vi "Flatten.vi"(6 "Persistence in":refnum<class "IPersist.lvclass">, 7 "Linked List Ref":refnum<data-value>, 8 "error in (no error)":errorcluster, 9 "Indent":i32, 10 "Active Unique ID":string, 11 "Executioner in":refnum<class "Executioner.lvclass">) -> (0 "error out":errorcluster, 2 "Active Unique ID out":string, 3 "Flattened Test Executive":string[](array[string]), 4 "Persistence out":refnum<class "IPersist.lvclass">, 5 "Linked List Ref out":refnum<data-value>)   [LabVIEW 2017, in "Test Executive.lvlib" / "Executioner.lvclass"]
uses:
  <vilib>/gpm_packages/@cs/test-executive/Source/Test Executive/Executioner/Executioner.lvclass
  <vilib>/gpm_packages/@cs/linked-list/Source/Linked List/ILinkedList/ILinked List.lvclass
  <vilib>/gpm_packages/@cs/persistence/source/IPersist/IPersist.lvclass
  <vilib>/gpm_packages/@cs/linked-list/Source/Linked List/Linked List Ref/Linked List Ref.lvclass
  <vilib>/gpm_packages/@cs/linked-list/Source/String Manipulation/String Manipulation.lvlib
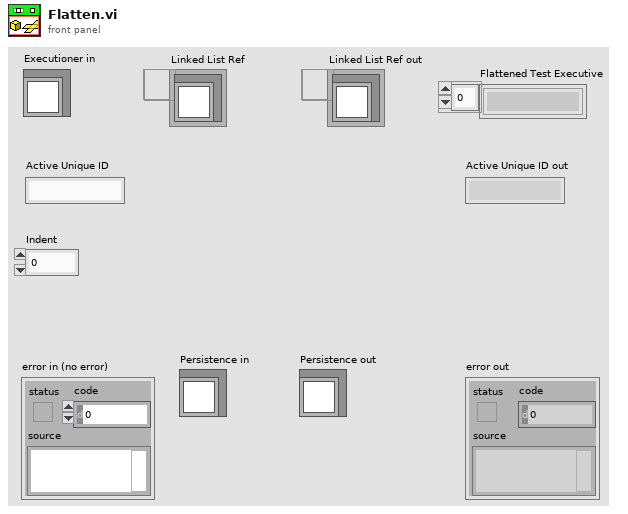
[diagram p1: front panel]
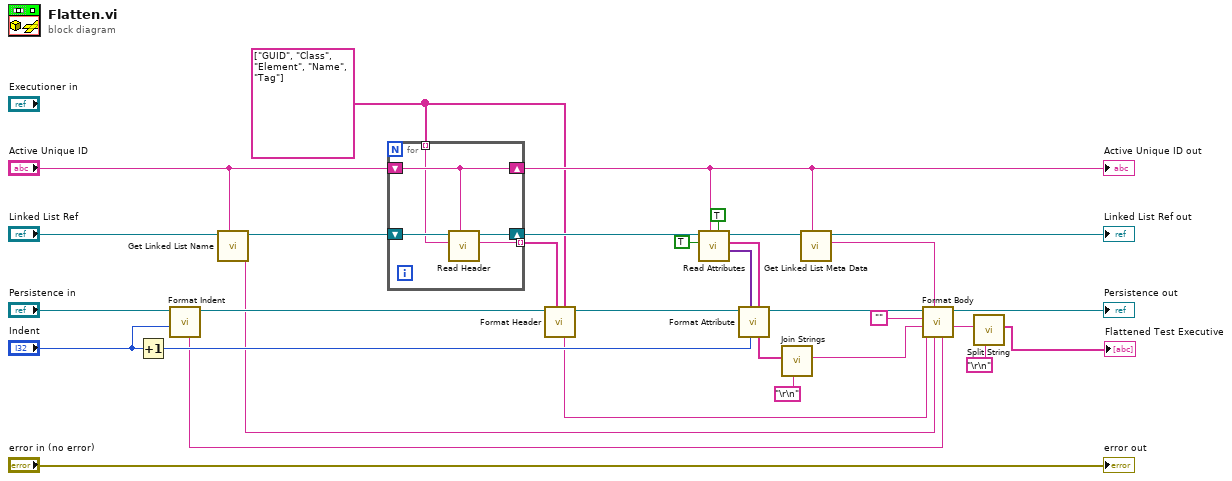
[diagram p0: block diagram]
diagram:
  w3 = string[] ["GUID", "Class", "Element", "Name", "Tag"]
  n1 = Increment(x="Indent") -> (x+1=w19:i32)
  n2 = call-dynamic "Format Indent.vi"("Indent"="Indent", "IPersist in"="Persistence in") -> ("IPersist out"=w30:refnum<class "IPersist.lvclass">, "Indent XML"=w15:string)  [unwired: 7 in, 1 out]
  n3 = call <vilib>:"Get Linked List Name.vi"("Linked List ID"="Active Unique ID", "Linked List Ref"="Linked List Ref") -> ("Linked List Name"=w14:string, "Linked List Ref out"=w28:refnum<data-value>)  [unwired: 6 in, 2 out]
  n4 = for {
    shift-right: [w36] -> w27
    shift-left: w28 -> [w37]
    shift-right: [w35] -> w4
    shift-left: "Active Unique ID" -> [w35]
    tunnel: w3 -> [w34] mode=indexing
    tunnel: [w33] -> w2 mode=indexing
    n5 = call <vilib>:"Read Header.vi"("Linked List ID"=w35, "Header Name"=w34, "Linked List Ref"=w37) -> ("Header Value"=w33:string, "Linked List Ref out"=w36:refnum<data-value>)  [unwired: 5 in, 2 out]
  }
  "Active Unique ID out" <- w4
  n6 = call-dynamic "Format Header.vi"("Name"=w3, "Value"=w2, "IPersist in"=w30) -> ("IPersist out"=w24:refnum<class "IPersist.lvclass">, "Header"=w10:string)  [unwired: 7 in]
  n7 = call <vilib>:"Read Attributes.vi"("Flatten Pointer?"=TRUE, "Linked List ID"=w4, "Include Private?"=TRUE, "Linked List Ref"=w27) -> ("Attributes"=w22:variant[], "Attribute Names out"=w21:string[], "Linked List Ref out"=w26:refnum<data-value>)  [unwired: 2 in, 3 out]
  n8 = call-dynamic "Format Attribute.vi"("Attribute Names"=w21, "Indent"=w19, "Attribute Values"=w22, "IPersist in"=w24) -> ("IPersist out"=w18:refnum<class "IPersist.lvclass">, "Attr Strings"=w12:string[])  [unwired: 6 in]
  n9 = call <vilib>:"Join Strings.vi"("Separator (,)"="\r\n", "Strings In"=w12) -> ("String"=w11:string)  [unwired: 9 in]
  n10 = call <vilib>:"Get Linked List Meta Data.vi"("Linked List ID"=w4, "Linked List Ref"=w26) -> ("Meta Data"=w16:string, "Linked List Ref out"=→"Linked List Ref out":refnum<data-value>)  [unwired: 6 in, 2 out]
  n11 = call-dynamic "Format Body.vi"("Indent"=w15, "Name"=w14, "Meta Data"=w16, "Header"=w10, "Attributes"=w11, "Body"="", "IPersist in"=w18) -> ("String out"=w7:string, "IPersist out"=→"Persistence out":refnum<class "IPersist.lvclass">)  [unwired: 3 in]
  n12 = call <vilib>:"Split String.vi"("Split Pattern"="\r\n", "Input String"=w7) -> ("Split String"=→"Flattened Test Executive":string[])  [unwired: 9 in]
  "error out" <- "error in (no error)"
